vi "Set_PScontrol.vi"(7 "Magnet PS":u16(ring) items=["Resistive Magnet", "SCM2", "SCM1"], 8 "error in (no error)":errorcluster, 10 "Command_Message_in":T2, 11 "Command_queue_in":T1) -> (0 "error out":errorcluster, 2 "Command_Message_out":T2, 3 "Command_queue_out":T1)   [LabVIEW 2019]
uses:
  Command_Message.ctl
  Command_Queue.ctl
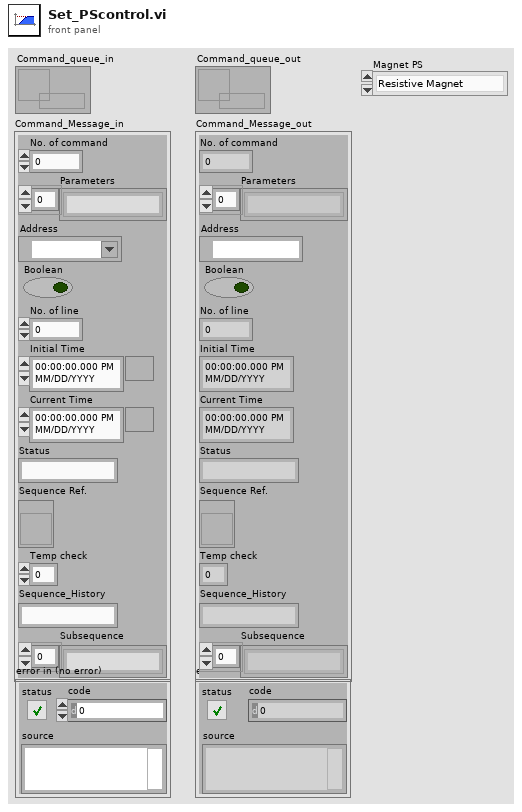
[diagram p1: front panel]
types:
  T1 = typedef "Command_Queue.ctl" = refnum<queue>
  T2 = typedef "Command_Message.ctl" = cluster{"No. of command":i32, "Parameters":string[], "Address":refnum<visa-resource-name>, "Boolean":bool, "No. of line":i32, "Initial Time":timestamp, "Current Time":timestamp, "Status":string, "Sequence Ref.":refnum<vi>, "Temp check":i32, "Sequence_History":string, "Subsequence":string[]}
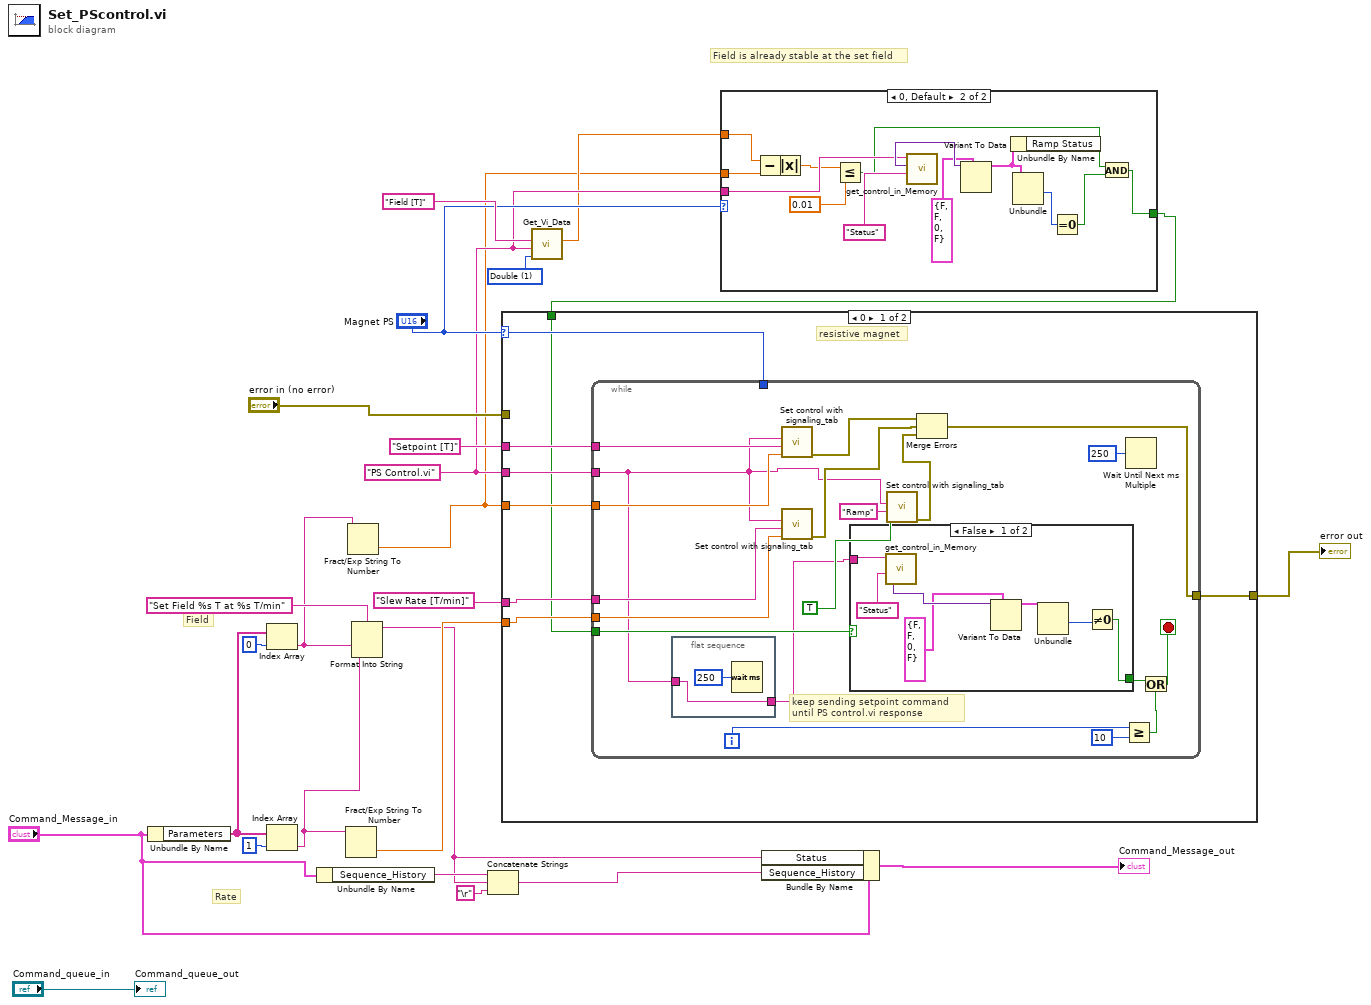
[diagram p0: block diagram]
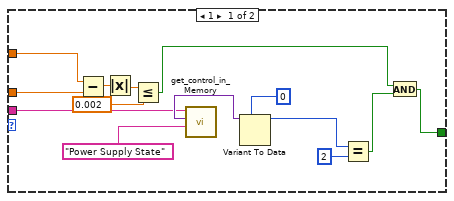
[diagram p2: hidden frame]
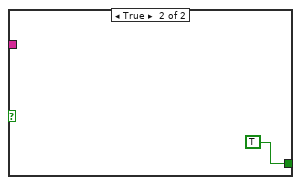
[diagram p3: hidden frame]
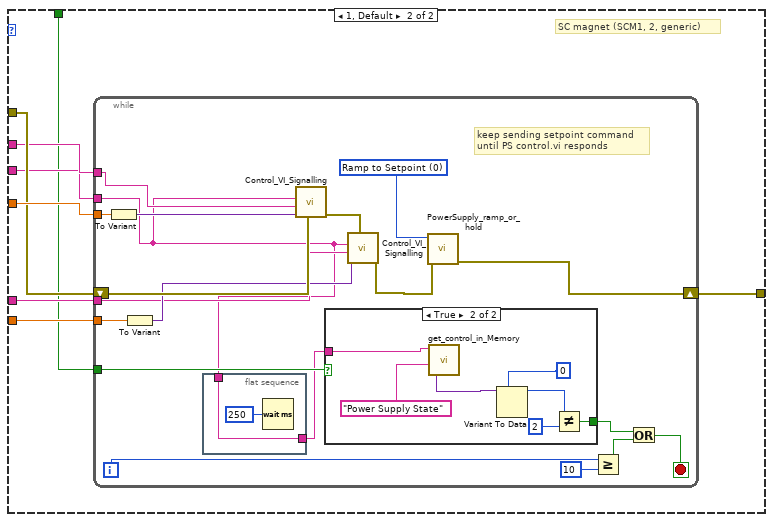
[diagram p4: hidden frame]
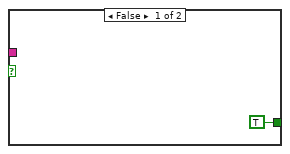
[diagram p5: hidden frame]
diagram:
  w5 = u16 1 items=["String", "Double", "Boolean", "Variant"] ("Data Type")
  w4 = "PS Control.vi" ("Target VI name")
  # "Field is already stable at the set field"
  # "Rate"
  # "Field"
  n1 = Unbundle By Name("Command_Message_in") -> ("Parameters"=w16:string[])
  n2 = Index Array(array=w16, index=0) -> (element=w19:string)
  n3 = Index Array(array=w16, index=1) -> (element=w18:string)
  n4 = Unbundle By Name("Command_Message_in") -> ("Sequence_History"=w13:string)
  n5 = Fract/Exp String To Number(string=w18) -> (number=w22:dbl)  [unwired: 3 in, 1 out]
  n6 = Fract/Exp String To Number(string=w19) -> (number=w2:dbl)  [unwired: 3 in, 1 out]
  n7 = Format Into String(format string="Set Field %s T at %s T/min", w19, w18) -> (resulting string=w12:string)  [unwired: 2 in, 1 out]
  n8 = Concatenate Strings(w13, w12, "\r") -> (w10:string)
  n9 = call "Get_Vi_Data.vi"("Data Type"=w5, "VI name"=w4, "Control Name"="Field [T]") -> ("Data (Double)"=w3:dbl)  [unwired: 4 in, 4 out]
  n10 = case shown="0, Default" "Magnet PS" {
    tunnel: w4 -> [w36 w51]
    tunnel: [w32 w50] -> w1
    tunnel: w3 -> [w31 w49]
    tunnel: w2 -> [w30 w48]
    frame 1 {
      n11 = Subtract(x=w31, y=w30) -> (x-y=w29:dbl)
      n12 = Absolute Value(x=w29) -> (abs(x)=w26:dbl)
      n13 = Less Or Equal?(x=w26, y=0.002) -> (x <= y?=w27:bool)
      n14 = call "get_control_in_Memory.vi"("Control Name"="Power Supply State", "VI Name"=w36) -> ("Value"=w38:variant)  [unwired: 2 in, 1 out]
      n15 = Variant To Data(type=0, Variant=w38) -> (data=w34:i32)  [unwired: 1 in, 1 out]
      n16 = Equal?(x=w34, y=2) -> (x = y?=w33:bool)
      n17 = And(x=w27, y=w33) -> (x .and. y?=w32:bool)
    }
    frame 0, Default {
      n18 = Subtract(x=w49, y=w48) -> (x-y=w47:dbl)
      n19 = Absolute Value(x=w47) -> (abs(x)=w43:dbl)
      n20 = Less Or Equal?(x=w43, y=0.01) -> (x <= y?=w45:bool)
      n21 = call "get_control_in_Memory.vi"("Control Name"="Status", "VI Name"=w51) -> ("Value"=w52:variant)  [unwired: 2 in, 1 out]
      n22 = Variant To Data(type=cluster{bool, bool, "Ramp Status":u16, bool} {FALSE, FALSE, "Ramp Status"=0, FALSE} ("Status"), Variant=w52) -> (data=w42:cluster{bool, bool, "Ramp Status":u16, bool})  [unwired: 1 in, 1 out]
      n23 = Unbundle By Name(w42) -> ()  [unwired: 1 out]
      n24 = Unbundle(w42) -> ("Ramp Status"=w41:u16)  [unwired: 3 out]
      n25 = Equal To 0?(x=w41) -> (x = 0?=w40:bool)
      n26 = And(x=w45, y=w40) -> (x .and. y?=w50:bool)
    }
  }
  n27 = case shown="0" "Magnet PS" {
    selector: "Magnet PS" -> [w55 _]
    tunnel: w2 -> [w57 w98]
    tunnel: "error in (no error)" -> [_ w97]
    tunnel: w22 -> [w56 w96]
    tunnel: [w61 w95] -> w21
    tunnel: "Setpoint [T]" -> [w60 w94]
    tunnel: w4 -> [w59 w92]
    tunnel: "Slew Rate [T/min]" ("Control Name") -> [w58 w93]
    tunnel: w1 -> [w54 w91]
    frame 0 {
      # "resistive magnet"
      n28 = while {
        tunnel: [w65] -> w61
        tunnel: w60 -> [w75]
        tunnel: w59 -> [w63]
        tunnel: w58 -> [w74]
        tunnel: w57 -> [w73]
        tunnel: w56 -> [w72]
        tunnel: w55 -> [_]
        tunnel: w54 -> [w64]
        i -> [w70]
        stop <- w66 stop-if-true
        # "keep sending setpoint command\nuntil PS control.vi response"
        n29 = flat-sequence {
          tunnel: [w81] -> w62
          tunnel: w63 -> [w81]
          frame #0 {
            n30 = Wait (ms)(milliseconds to wait=u32 250) -> ()  [unwired: 1 out]
          }
        }
        n31 = call "Set control with signaling_tab.vi"("Value (Signaling)"=w73, "Control Name"=w75, "VI Name"=w63) -> ("error out"=w78:errorcluster)  [unwired: 8 in]
        n32 = call "Set control with signaling_tab.vi"("Value (Signaling)"=w72, "Control Name"=w74, "VI Name"=w63) -> ("error out"=w77:errorcluster)  [unwired: 8 in]
        n33 = case shown="False" w64 {
          tunnel: w62 -> [w84 _]
          tunnel: [w83 TRUE] -> w68
          frame False {
            n34 = call "get_control_in_Memory.vi"("Control Name"="Status", "VI Name"=w84) -> ("Value"=w88:variant)  [unwired: 2 in, 1 out]
            n35 = Variant To Data(type=cluster{bool, bool, "Ramp Status":u16, bool} {FALSE, FALSE, "Ramp Status"=0, FALSE} ("Status"), Variant=w88) -> (data=w89:cluster{bool, bool, "Ramp Status":u16, bool})  [unwired: 1 in, 1 out]
            n36 = Unbundle(w89) -> ("Ramp Status"=w85:u16)  [unwired: 3 out]
            n37 = Not Equal To 0?(x=w85) -> (x != 0?=w83:bool)
          }
          frame True {
          }
        }
        n38 = call "Set control with signaling_tab.vi"("Value (Signaling)"=TRUE, "Control Name"="Ramp", "VI Name"=w63) -> ("error out"=w76:errorcluster)  [unwired: 8 in]
        n39 = Merge Errors(w78, w77, w76) -> (w65:errorcluster)
        n40 = Greater Or Equal?(x=w70, y=10) -> (x >= y?=w67:bool)
        n41 = Wait Until Next ms Multiple(millisecond multiple=u32 250) -> ()  [unwired: 1 out]
        n42 = Or(x=w68, y=w67) -> (x .or. y?=w66:bool)
      }
    }
    frame 1, Default {
      # "SC magnet (SCM1, 2, generic)"
      n43 = while {
        tunnel: w98 -> [w117]
        tunnel: w96 -> [w113]
        tunnel: w94 -> [w108]
        tunnel: w92 -> [w99]
        tunnel: w93 -> [w107]
        shift-right: [w109] -> w95
        shift-left: w97 -> [w115]
        tunnel: w91 -> [w101]
        i -> [w106]
        stop <- w102 stop-if-true
        w110 = u16 0 items=["Ramp to Setpoint", "Hold"] ("Mode")
        # "keep sending setpoint command\nuntil PS control.vi responds"
        n44 = To Variant(anything=w117) -> (Variant=w116:variant)
        n45 = To Variant(anything=w113) -> (Variant=w112:variant)
        n46 = flat-sequence {
          tunnel: [w118] -> w100
          tunnel: w99 -> [w118]
          frame #0 {
            n47 = Wait (ms)(milliseconds to wait=u32 250) -> ()  [unwired: 1 out]
          }
        }
        n48 = call "Control_VI_Signalling.vi"("error in (no error)"=w115, "Input Value"=w116, "Control Name"=w108, "Target VI name"=w99) -> ("error out"=w114:errorcluster)  [unwired: 7 in]
        n49 = case shown="True" w101 {
          tunnel: [TRUE w122] -> w104
          tunnel: w100 -> [_ w121]
          frame False {
          }
          frame True {
            n50 = call "get_control_in_Memory.vi"("Control Name"="Power Supply State", "VI Name"=w121) -> ("Value"=w126:variant)  [unwired: 2 in, 1 out]
            n51 = Variant To Data(type=0, Variant=w126) -> (data=w124:i32)  [unwired: 1 in, 1 out]
            n52 = Not Equal?(x=w124, y=2) -> (x != y?=w122:bool)
          }
        }
        n53 = call "Control_VI_Signalling.vi"("error in (no error)"=w114, "Input Value"=w112, "Control Name"=w107, "Target VI name"=w99) -> ("error out"=w111:errorcluster)  [unwired: 7 in]
        n54 = call "PowerSupply_ramp_or_hold.vi"("error in (no error)"=w111, "Mode"=w110) -> ("error out"=w109:errorcluster)  [unwired: 9 in]
        n55 = Greater Or Equal?(x=w106, y=10) -> (x >= y?=w103:bool)
        n56 = Or(x=w104, y=w103) -> (x .or. y?=w102:bool)
      }
    }
  }
  "error out" <- w21
  n57 = Bundle By Name(cluster="Command_Message_in", "Status"=w12, "Sequence_History"=w10) -> (→"Command_Message_out":T2)
  "Command_queue_out" <- "Command_queue_in"
